vi "Initialize.vi"(7 "Serial Configuration":T1={"Baud Rate"=9600, "Parity"=0, "Data Bits"=8, "Stop Bits"=10, "Flow Control"=0} {"Flow Control" items=["None", "XON/XOFF", "RTS/CTS", "XON/XOFF & RTS/CTS", "DTR/DSR", "XON/XOFF & DTR/DSR"]; "Stop Bits" items=["1.0"=10, "1.5"=15, "2.0"=20]; "Data Bits" items=["7"=7, "8"=8]; "Parity" items=["None", "Odd", "Even", "Mark", "Space"]; "Baud Rate" items=["300"=300, "600"=600, "1200"=1200, "2400"=2400, "4800"=4800, "9600"=9600, "19200"=19200]}, 8 "error in (no error)":errorcluster, 9 "Reset (True)":bool, 10 "ID Query (True)":bool, 11 "VISA resource name":refnum<visa-resource-name>) -> (0 "error out":errorcluster, 3 "VISA resource name out":refnum<visa-resource-name>)   [LabVIEW 2015, in "IT6700H.lvlib"]
doc: "Establishes communication with the instrument and optionally performs an instrument identification query and/or an instrument reset. It also places the instrument in a default state needed for other instrument driver operations. Therefore, call this VI before calling other instrument driver VIs for this instrument. Generally, you need to call the <b>Initialize</b> VI only once at the beginning of an application."
uses:
  <instrlib>/IT6700H/IT6700H.lvlib
panel:
  # "(c) 2014 <Enter Company Name Here>.  ALL RIGHTS RESERVED."
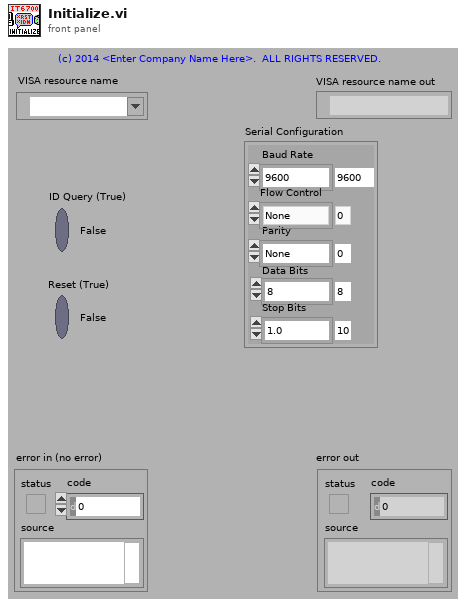
[diagram p1: front panel]
types:
  T1 = cluster{"Baud Rate":u32, "Parity":u16, "Data Bits":u16, "Stop Bits":u16, "Flow Control":u16}
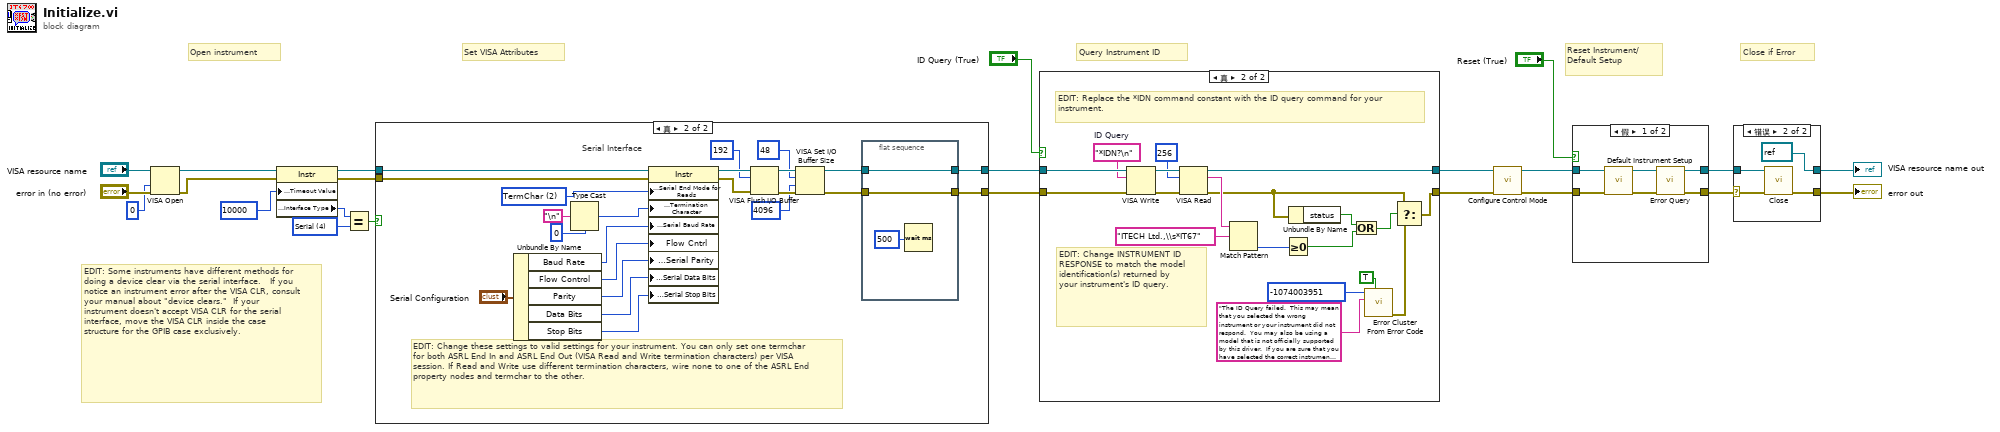
[diagram p0: block diagram]
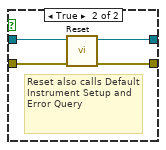
[diagram p4: hidden frame]
diagram:
  w12 = u16 4 items=["GPIB"=1, "VXI"=2, "GPIB-VXI"=3, "Serial"=4, "PXI"=5, "TCPIP"=6, "USB"=7] ("Interface Information:Interface Type")
  # "EDIT: Some instruments have different methods for doing a device clear via the serial interface.   If you notice an instrument error after the VISA CLR, consult your manual about \"device clears.\"  If your instrument doesn't accept VISA CLR for the serial interface, move the VISA CLR inside the case  structure for the GPIB case exclusively."
  # "Set VISA Attributes"
  # "Close if Error"
  # "Query Instrument ID"
  # "Reset Instrument/\nDefault Setup"
  # "Open instrument"
  n1 = VISA Open(access mode=u32 0, error in (no error)="error in (no error)", VISA resource name="VISA resource name") -> (VISA resource name=w6:refnum<visa-resource-name>, error out=w5:errorcluster)  [unwired: 2 in]
  n2 = property class="Instr"(reference=w6, error in=w5, "General Settings:Timeout Value"=u32 10000) -> (reference out=w15:refnum<visa-resource-name>, error out=w14:errorcluster, "Interface Information:Interface Type"=w19:u16)
  n3 = Equal?(x=w19, y=w12) -> (x = y?=w13:bool)
  n4 = case shown="真" w13 {
    tunnel: [w24 w28] -> w17
    tunnel: [w25 w26] -> w16
    tunnel: w15 -> [w24 w32]
    tunnel: w14 -> [w25 w31]
    frame False {
      # "EDIT: Remove interfaces not supported by your instrument."
      # "GPIB, TCP/IP, and USB Interface"
    }
    frame True {
      w39 = u16 2 items=["None", "LastBit", "TermChar"] ("Serial Settings:Serial End Mode for Reads")
      # "EDIT: Change these settings to valid settings for your instrument. You can only set one termchar for both ASRL End In and ASRL End Out (VISA Read and Write termination characters) per VISA session. If Read and Write use different termination characters, wire none to one of the ASRL End property nodes and termchar to the other."
      # "Serial Interface"
      n5 = Unbundle By Name("Serial Configuration") -> ("Baud Rate"=w37:u32, "Flow Control"=w30:u16, "Parity"=w35:u16, "Data Bits"=w36:u16, "Stop Bits"=w33:u16)
      n6 = Type Cast(type=u8 0, x="\n" ("Line Feed Constant")) -> (*(type *) &x=w38:u8)
      n7 = property class="Instr"(reference=w32, error in=w31, "Serial Settings:Serial End Mode for Reads"=w39, "Message Based Settings:Termination Character"=w38, "Serial Settings:Serial Baud Rate"=w37, "Flow Cntrl"=w30, "Serial Settings:Serial Parity"=w35, "Serial Settings:Serial Data Bits"=w36, "Serial Settings:Serial Stop Bits"=w33) -> (reference out=w45:refnum<visa-resource-name>, error out=w47:errorcluster)
      n8 = VISA Flush I/O Buffer(VISA resource name=w45, mask (16)=u16 192, error in (no error)=w47) -> (VISA resource name out=w48:refnum<visa-resource-name>, error out=w46:errorcluster)
      n9 = VISA Set I/O Buffer Size(VISA resource name=w48, mask (16)=u16 48, size (4096)=u32 4096 ("size (0)"), error in (no error)=w46) -> (VISA resource name out=w29:refnum<visa-resource-name>, error out=w27:errorcluster)
      n10 = flat-sequence {
        tunnel: w29 -> [w51]
        tunnel: [w51] -> w28
        tunnel: w27 -> [w50]
        tunnel: [w50] -> w26
        frame #0 {
          n11 = Wait (ms)(milliseconds to wait=500) -> ()  [unwired: 1 out]
        }
      }
    }
  }
  n12 = case shown="真" "ID Query (True)" {
    tunnel: [w52 w72] -> w4
    tunnel: [w53 w69] -> w3
    tunnel: w17 -> [w53 w70]
    tunnel: w16 -> [w52 w71]
    frame False {
    }
    frame True {
      w63 = "*IDN?\n"  # ID Query
      # "EDIT: Replace the *IDN command constant with the ID query command for your instrument."
      # "EDIT: Change INSTRUMENT ID RESPONSE to match the model identification(s) returned by your instrument's ID query."
      n13 = VISA Write(VISA resource name=w70, write buffer=w63, error in (no error)=w71) -> (VISA resource name out=w67:refnum<visa-resource-name>, error out=w66:errorcluster)  [unwired: 1 out]
      n14 = VISA Read(VISA resource name=w67, byte count=u32 256, error in (no error)=w66) -> (VISA resource name out=w69:refnum<visa-resource-name>, read buffer=w68:string, error out=w57:errorcluster)  [unwired: 1 out]
      n15 = Match Pattern(string=w68, regular expression="ITECH Ltd.,\\s*IT67") -> (offset past match=w58:i32)  [unwired: 1 in, 3 out]
      n16 = Greater Or Equal To 0?(x=w58) -> (x >= 0?=w55:bool)
      n17 = Unbundle By Name(w57) -> ("status"=w56:bool)
      n18 = Or(x=w56, y=w55) -> (x .or. y?=w54:bool)
      n19 = call <vilib>:"Error Cluster From Error Code.vi"("show call chain? (False)"=TRUE, "error message (\"\")"="The ID Query failed.  This may mean that you selected the wrong instrument or your instrument did not respond.  You may also be using a model that is not officially supported by this driver.  If you are sure that you have selected the correct instrument and it is responding, try disabling the ID Query." ("Source (VI Name)"), "error code (0)"=-1074003951 ("Code")) -> ("error out"=w62:errorcluster)  [unwired: 6 in]
      n20 = Select(t=w57, s=w54, f=w62) -> (s? t:f=w72:errorcluster)
    }
  }
  n21 = call <instrlib>:"Configure Control Mode.vi"("error in (no error)"=w4, "VISA resource name"=w3) -> ("error out"=w1:errorcluster, "VISA resource name out"=w2:refnum<visa-resource-name>)  [unwired: 8 in]
  n22 = case shown="假" "Reset (True)" {
    tunnel: w1 -> [w73 w79]
    tunnel: [w77 w82] -> w7
    tunnel: w2 -> [w74 w80]
    tunnel: [w78 w81] -> w8
    frame False {
      n23 = call <instrlib>:"Default Instrument Setup.vi"("error in (no error)"=w73, "VISA resource name"=w74) -> ("error out"=w76:errorcluster, "VISA resource name out"=w75:refnum<visa-resource-name>)  [unwired: 8 in]
      n24 = call <instrlib>:"Error Query.vi"("error in (no error)"=w76, "VISA resource name"=w75) -> ("error out"=w77:errorcluster, "VISA resource name out"=w78:refnum<visa-resource-name>)  [unwired: 6 in, 2 out]
    }
    frame True {
      # "Reset also calls Default Instrument Setup and Error Query"
      n25 = call <instrlib>:"Reset.vi"("error in (no error)"=w79, "VISA resource name"=w80) -> ("error out"=w82:errorcluster, "VISA resource name out"=w81:refnum<visa-resource-name>)  [unwired: 8 in]
    }
  }
  n26 = case shown="错误" w7 {
    selector: w7 -> [w83 w86]
    tunnel: w8 -> [w84 w87]
    tunnel: [w84 refnum<visa-resource-name> refnum ("VISA resource name out")] -> w10
    tunnel: [w83 w88] -> w9
    frame No Error {
    }
    frame Error {
      n27 = call <instrlib>:"Close.vi"("error in (no error)"=w86, "VISA resource name"=w87) -> ("error out"=w88:errorcluster)  [unwired: 9 in]
    }
  }
  "VISA resource name out" <- w10
  "error out" <- w9
